vi "get runtime class name.vi"(8 "error in":errorcluster, 11 "configuration in":refnum<class "TBM configuration.lvclass">) -> (0 "error out":errorcluster, 2 "class name":string, 3 "configuration out":refnum<class "TBM configuration.lvclass">)   [LabVIEW 2013, in "TBM configuration.lvclass"]
doc: "Provides an interface for determining the runtime class associated with this configuration. This class name can then be used to dynamically load or locate the runtime class for initialization purposes."
uses:
  TBM configuration.lvclass
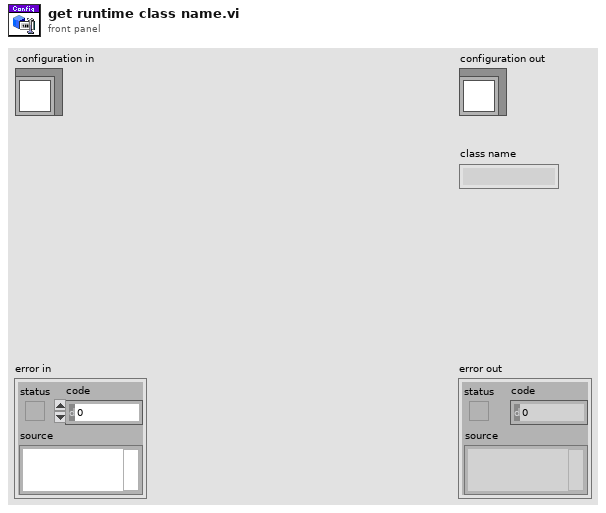
[diagram p1: front panel]
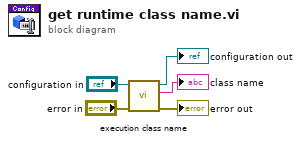
[diagram p0: block diagram]
diagram:
  n1 = call-dynamic "execution class name.vi"("error in"="error in", "configuration in"="configuration in") -> ("error out"=→"error out":errorcluster, "execution class"=→"class name":string, "configuration out"=→"configuration out":refnum<class "TBM configuration.lvclass">)  [unwired: 7 in]
